vi "Remove Entry.vi"(10 "Source":string, 11 "Message History in":string[][](array[string])) -> (3 "Message History out":string[][](array[string]))   [LabVIEW 2020]
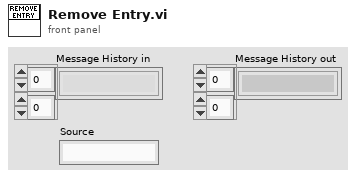
[diagram p1: front panel]
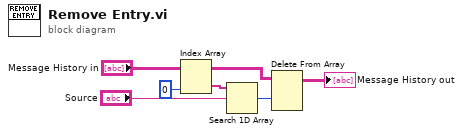
[diagram p0: block diagram]
diagram:
  n1 = Index Array(array="Message History in", index (col)=0 ("disabled index (col)")) -> (element=w3:string[])  [unwired: 1 in]
  n2 = Search 1D Array(1D array=w3, element="Source") -> (index of element=w1:i32)  [unwired: 1 in]
  n3 = Delete From Array(array="Message History in", index (row)=w1) -> (array with subset deleted=→"Message History out":string[][])  [unwired: 2 in, 1 out]
